vi "STS_Connect.vi"(8 "error in":errorcluster, 11 "Address Cluster out输入":T1 {"tsl_communcation_method" items=["GPIB", "C232C", "TCPIP", "USB"]; "MPM_communcation_method" items=["GPIB", "C232C", "TCPIP", "USB"]}) -> (0 "error out":errorcluster, 3 "Address Cluster out":T1 {"tsl_communcation_method" items=["GPIB", "C232C", "TCPIP", "USB"]; "MPM_communcation_method" items=["GPIB", "C232C", "TCPIP", "USB"]})   [LabVIEW 2017]
uses:
  CTL/Address Cluster.ctl
  D:/test/ILSTS/LV_IL/LV_IL_Sample_x86/DLL/InstrumentDLL.dll
  DLL/InstrumentDLL.dll
  Share/PowerMonitorType.vi
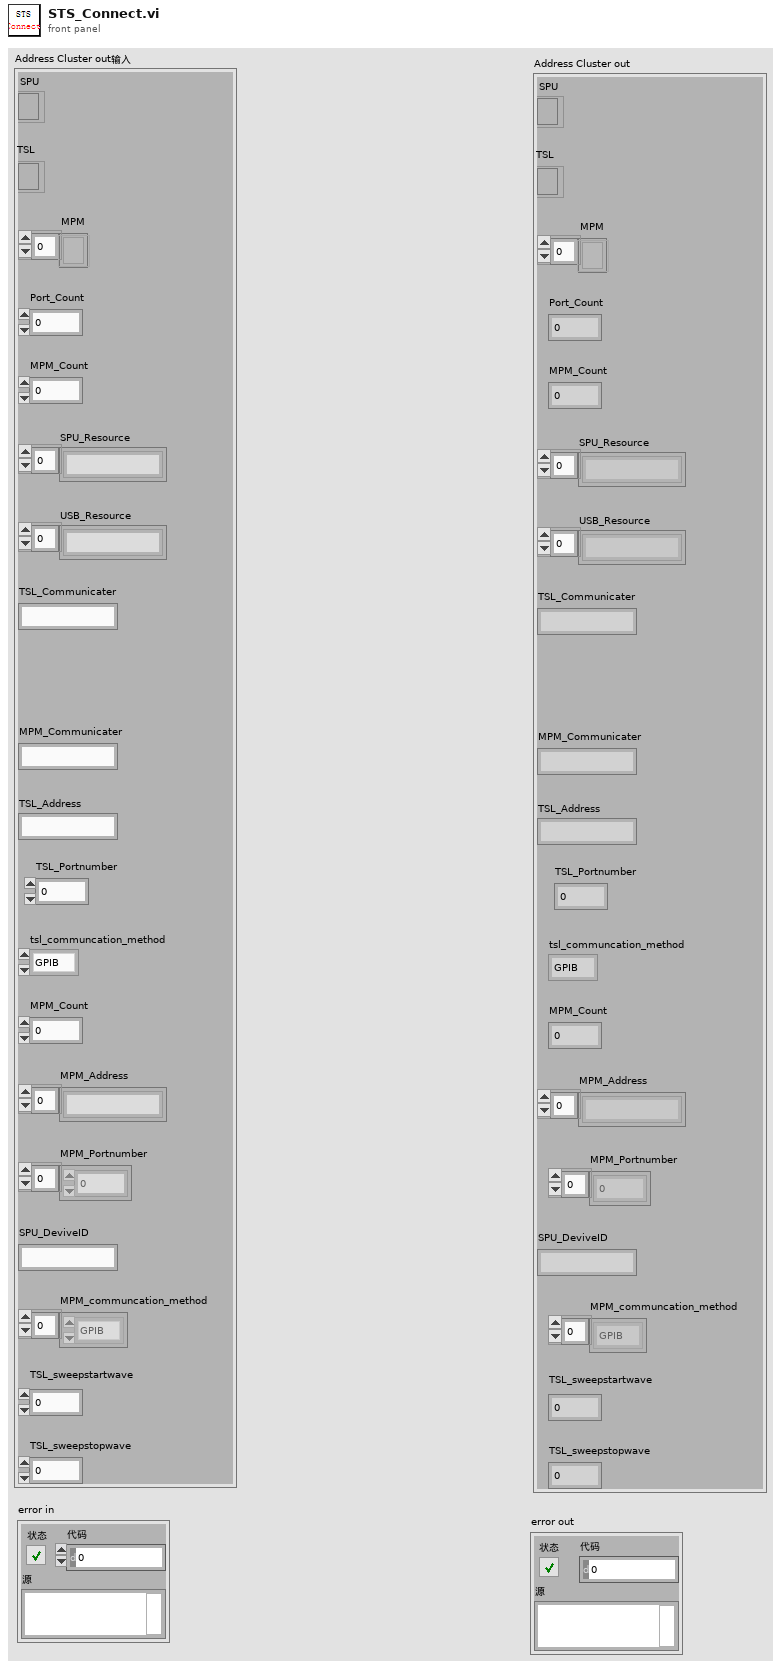
[diagram p1: front panel]
types:
  T1 = typedef "Address Cluster.ctl" = cluster{"SPU":refnum<k24>, "MPM":refnum<k24>[], "Port_Count":dbl, "MPM_Count":dbl, "SPU_Resource":string[], "USB_Resource":string[], "MPM_Communicater":string, "MPM_Count":dbl, "MPM_Address":string[], "MPM_Portnumber":dbl[], "SPU_DeviveID":string, "MPM_communcation_method":i32[], "TSL_sweepstartwave":dbl, "TSL_sweepstopwave":dbl, "TSL_Address":string, "TSL_Communicater":string, "TSL":refnum<k24>, "tsl_communcation_method":i32, "TSL_Portnumber":dbl}
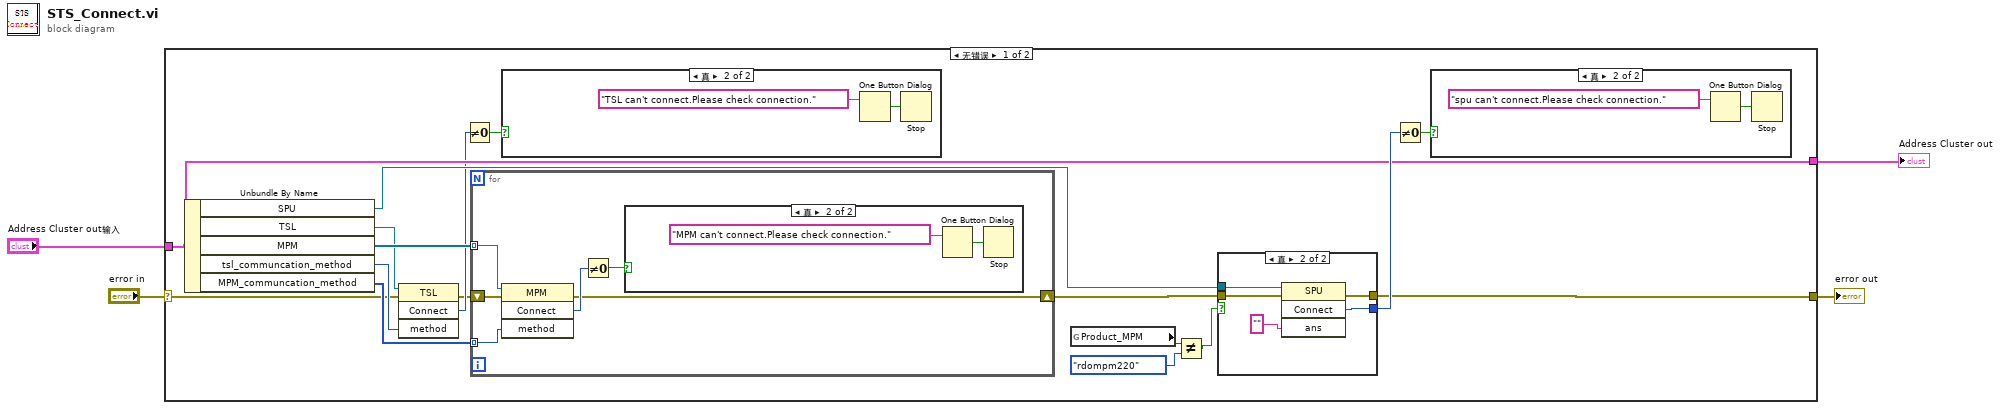
[diagram p0: block diagram]
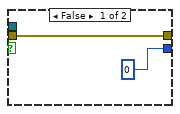
[diagram p2: hidden frame]
diagram:
  n1 = case shown="无错误" "error in" {
    selector: "error in" -> [w14 w42]
    tunnel: "Address Cluster out输入" -> [w13 w41]
    tunnel: [w8 w42] -> w2
    tunnel: [w13 w41] -> w1
    frame No Error {
      n2 = Unbundle By Name(w13) -> ("SPU"=w19:refnum<k24>, "TSL"=w15:refnum<k24>, "MPM"=w17:refnum<k24>[], "tsl_communcation_method"=w16:i32, "MPM_communcation_method"=w18:i32[])
      n3 = invoke on="调用节点" class="TSL" method="Connect"(reference=w15, error in=w14, "method"=w16) -> (error out=w10:errorcluster, "Connect"=w12:i32)  [unwired: 1 in, 2 out]
      n4 = Not Equal To 0?(x=w12) -> (x != 0?=w11:bool)
      n5 = for {
        tunnel: w17 -> [w38] mode=indexing
        tunnel: w18 -> [w37] mode=indexing
        shift-right: [w34] -> w9
        shift-left: w10 -> [w33]
        n6 = invoke on="调用节点" class="MPM" method="Connect"(reference=w38, error in=w33, "method"=w37) -> (error out=w34:errorcluster, "Connect"=w35:i32)  [unwired: 1 in, 2 out]
        n7 = Not Equal To 0?(x=w35) -> (x != 0?=w36:bool)
        n8 = case shown="真" w36 {
          frame False {
          }
          frame True {
            n9 = One Button Dialog(message="MPM can't connect.Please check connection." ("消息")) -> (true=w39:bool)  [unwired: 1 in]
            n10 = Stop(stop? (T)=w39) -> ()
          }
        }
      }
      n11 = case shown="真" w11 {
        frame False {
        }
        frame True {
          n12 = One Button Dialog(message="TSL can't connect.Please check connection." ("消息")) -> (true=w29:bool)  [unwired: 1 in]
          n13 = Stop(stop? (T)=w29) -> ()
        }
      }
      n14 = global read "PowerMonitorType.vi" "Product_MPM"() -> (w7:enum32{"rdompm210", "rdompm220"})
      n15 = Not Equal?(x=w7, y=enum32{"rdompm210", "rdompm220"}."rdompm220") -> (x != y?=w6:bool)
      n16 = case shown="真" w6 {
        tunnel: [0 ("Connect") w28] -> w21
        tunnel: w19 -> [_ w27]
        tunnel: w9 -> [w23 w25]
        tunnel: [w23 w24] -> w8
        frame False {
        }
        frame True {
          n17 = invoke class="SPU" method="Connect"(reference=w27, error in=w25, "ans"="") -> (error out=w24:errorcluster, "Connect"=w28:i32)  [unwired: 1 in, 2 out]
        }
      }
      n18 = Not Equal To 0?(x=w21) -> (x != 0?=w20:bool)
      n19 = case shown="真" w20 {
        frame False {
        }
        frame True {
          n20 = One Button Dialog(message="spu can't connect.Please check connection." ("消息")) -> (true=w31:bool)  [unwired: 1 in]
          n21 = Stop(stop? (T)=w31) -> ()
        }
      }
    }
    frame Error {
    }
  }
  "Address Cluster out" <- w1
  "error out" <- w2
